vi "Create Engine Project.vi"(8 "error in":errorcluster, 10 "Custom Device Name":string, 11 "CDEW_MetaDataObj in":refnum<class "NIVS_CDEW_MetaDataObj.lvclass">) -> (0 "error out":errorcluster, 3 "CDEW_MetaDataObj out":refnum<class "NIVS_CDEW_MetaDataObj.lvclass">)   [LabVIEW 2026, in "NIVS_CDEW_MetaDataObj.lvclass"]
uses:
  NIVS_CDEW_MetaDataObj.lvclass
  Types/EngineProjectToolStates.ctl
  NIVS_CDEW_MetaDataObj.lvclass/NIVS_CDEW_MetaDataObj.ctl
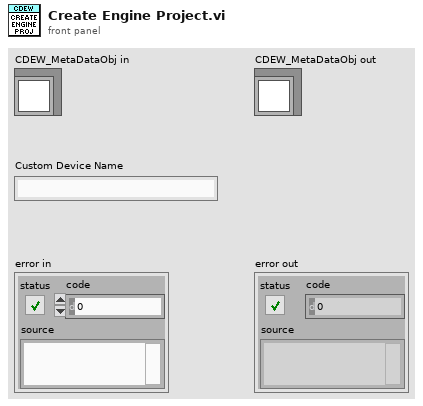
[diagram p1: front panel]
types:
  T1 = typedef "NIVS_CDEW_MetaDataObj.lvclass/EngineProjectToolStates.ctl" = enum16{"CreateEngineFolder", "CopyAndRenameEngineLVLIB", "UpdateLVLIBsInProject"}
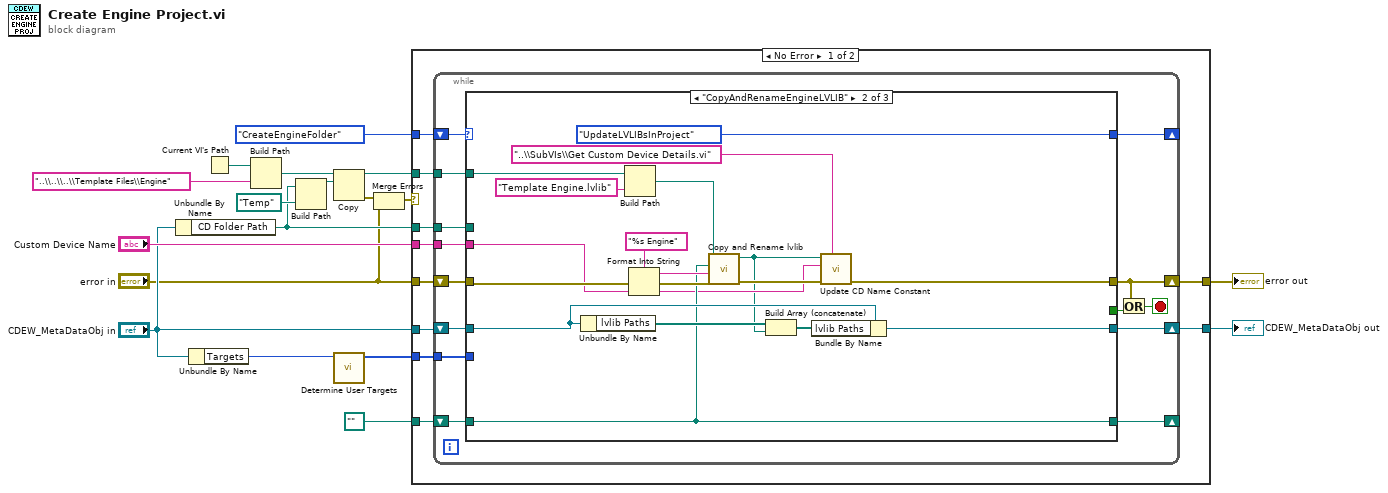
[diagram p0: block diagram]
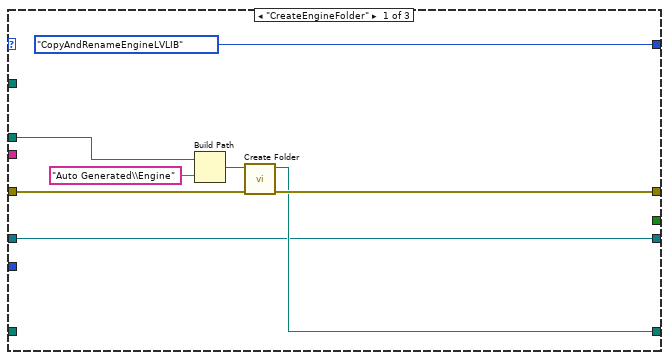
[diagram p2: hidden frame]
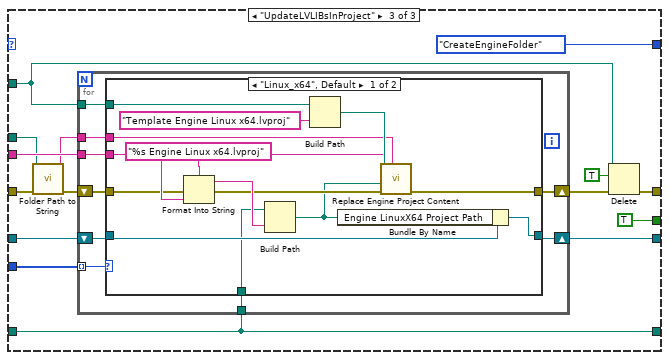
[diagram p3: hidden frame]
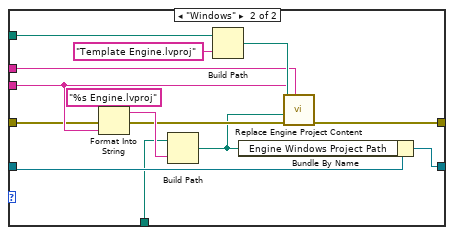
[diagram p4: hidden frame]
diagram:
  n1 = Unbundle By Name("CDEW_MetaDataObj in") -> ("CD Folder Path"=w8:path)
  n2 = Unbundle By Name("CDEW_MetaDataObj in") -> ("Targets"=w4:enum16{"Linux_x64", "Windows", "All"})
  n3 = Current VI's Path() -> (path=w16:path)
  n4 = Build Path(base path=w16, name or relative path="..\\..\\..\\Template Files\\Engine") -> (appended path=w11:path)
  n5 = Build Path(base path=w8, name or relative path=path "Temp") -> (appended path=w12:path)
  n6 = Copy(10:w12, 11:w11) -> (0:w3:errorcluster, 3:w10:path)  [unwired: 3 in, 1 out]
  n7 = call "Determine User Targets.vi"("Targets"=w4) -> ("User Configured Targets"=w5:enum16{"Linux_x64", "Windows", "All"}[])  [unwired: 10 in]
  n8 = Merge Errors(w3, "error in") -> (w1:errorcluster)
  n9 = case shown="No Error" w1 {
    selector: w1 -> [_ w120]
    tunnel: EngineProjectToolStates."CreateEngineFolder" -> [w28 _]
    tunnel: "Custom Device Name" -> [w27 _]
    tunnel: "error in" -> [w26 _]
    tunnel: [w25 w120] -> w14
    tunnel: w10 -> [w24 _]
    tunnel: [w23 w119] -> w9
    tunnel: w8 -> [w22 _]
    tunnel: path "" ("HarnessProjectPath") -> [w21 _]
    tunnel: "CDEW_MetaDataObj in" -> [w20 w119]
    tunnel: w5 -> [w19 _]
    frame No Error {
      n10 = while {
        shift-right: [w39] -> _
        shift-left: w28 -> [w42]
        tunnel: w27 -> [w41]
        tunnel: w24 -> [w40]
        shift-right: [w31] -> w23
        shift-left: w20 -> [w38]
        shift-right: [w36] -> w25
        shift-left: w26 -> [w37]
        shift-right: [w33] -> _
        shift-left: w21 -> [w32]
        tunnel: w22 -> [w30]
        tunnel: w19 -> [w29]
        stop <- w34 stop-if-true
        n11 = case shown="\"CopyAndRenameEngineLVLIB\"" w42 {
          tunnel: w41 -> [_ w53 w78]
          tunnel: w40 -> [_ w67 w72]
          tunnel: [EngineProjectToolStates."CopyAndRenameEngineLVLIB" EngineProjectToolStates."UpdateLVLIBsInProject" EngineProjectToolStates."CreateEngineFolder"] -> w39
          tunnel: [_ _ TRUE] -> w35
          tunnel: [w46 w57 w77] -> w31
          tunnel: w38 -> [w46 w59 w76]
          tunnel: [w48 w54 w80] -> w36
          tunnel: w37 -> [w49 w61 w69]
          tunnel: [w47 w56 w75] -> w33
          tunnel: w32 -> [_ w56 w75]
          tunnel: w30 -> [w45 _ w74]
          tunnel: w29 -> [_ _ w71]
          frame "CreateEngineFolder" {
            n12 = Build Path(base path=w45, name or relative path="Auto Generated\\Engine") -> (appended path=w44:path)
            n13 = call "Create Folder.vi"("error in"=w49, "Folder Path"=w44) -> ("error out"=w48:errorcluster, "Folder Path Out"=w47:path)  [unwired: 8 in]
          }
          frame "CopyAndRenameEngineLVLIB" {
            n14 = Unbundle By Name(w59) -> ("lvlib Paths"=w60:path[])
            n15 = Build Path(base path=w67, name or relative path="Template Engine.lvlib" ("string")) -> (appended path=w65:path)
            n16 = Format Into String(format string="%s Engine" ("string"), error in=w61, w53) -> (resulting string=w63:string, error out=w62:errorcluster)  [unwired: 1 in]
            n17 = call "Copy and Rename lvlib.vi"("error in"=w62, "New lvlib Name"=w63, "Destination Directory Path"=w56, "lvlib Path"=w65) -> ("error out"=w55:errorcluster, "New Library Path"=w52:path)  [unwired: 6 in]
            n18 = Build Array (concatenate)(w60, w52) -> (w58:path[])
            n19 = Bundle By Name(cluster=w59, "lvlib Paths"=w58) -> (w57:refnum<class "NIVS_CDEW_MetaDataObj.lvclass">)
            n20 = call "Update CD Name Constant.vi"("vi Name"="..\\SubVIs\\Get Custom Device Details.vi", "error in"=w55, "Custom Device Name"=w53, "lvlib Path"=w52) -> ("error out"=w54:errorcluster)  [unwired: 7 in]
          }
          frame "UpdateLVLIBsInProject" {
            n21 = call "Folder Path to String.vi"("error in"=w69, "CD Folder Path"=w74) -> ("error out"=w70:errorcluster, "Path as String"=w73:string)  [unwired: 8 in]
            n22 = for {
              tunnel: w72 -> [w91]
              tunnel: w78 -> [w90]
              tunnel: w75 -> [w86]
              tunnel: w73 -> [w85]
              shift-right: [w92] -> w81
              shift-left: w70 -> [w89]
              shift-right: [w88] -> w77
              shift-left: w76 -> [w87]
              tunnel: w71 -> [w84] mode=indexing
              n23 = case shown="\"Linux_x64\", Default" w84 {
                tunnel: [w103 w116] -> w92
                tunnel: w91 -> [w102 w115]
                tunnel: w90 -> [w101 w114]
                tunnel: w89 -> [w98 w111]
                tunnel: [w96 w109] -> w88
                tunnel: w87 -> [w95 w108]
                tunnel: w86 -> [w94 w107]
                tunnel: w85 -> [w93 w106]
                frame "Linux_x64", Default {
                  n24 = Format Into String(format string="%s Engine Linux x64.lvproj" ("Custom Device Name"), w101) -> (resulting string=w99:string)  [unwired: 2 in, 1 out]
                  n25 = Build Path(base path=w94, name or relative path=w99) -> (appended path=w97:path)
                  n26 = Build Path(base path=w102, name or relative path="Template Engine Linux x64.lvproj" ("Custom Device Name")) -> (appended path=w104:path)
                  n27 = Bundle By Name(cluster=w95, "Engine LinuxX64 Project Path"=w97) -> (w96:refnum<class "NIVS_CDEW_MetaDataObj.lvclass">)
                  n28 = call "Replace Engine Project Content.vi"("CDFolderPath String"=w93, "error in"=w98, "Custom Device Project Path"=w97, "CD Name"=w101, "Template Project path"=w104) -> ("error out"=w103:errorcluster)  [unwired: 6 in]
                }
                frame "Windows" {
                  n29 = Format Into String(format string="%s Engine.lvproj" ("Custom Device Name"), w114) -> (resulting string=w112:string)  [unwired: 2 in, 1 out]
                  n30 = Build Path(base path=w107, name or relative path=w112) -> (appended path=w110:path)
                  n31 = Build Path(base path=w115, name or relative path="Template Engine.lvproj" ("Custom Device Name")) -> (appended path=w117:path)
                  n32 = Bundle By Name(cluster=w108, "Engine Windows Project Path"=w110) -> (w109:refnum<class "NIVS_CDEW_MetaDataObj.lvclass">)
                  n33 = call "Replace Engine Project Content.vi"("CDFolderPath String"=w106, "error in"=w111, "Custom Device Project Path"=w110, "CD Name"=w114, "Template Project path"=w117) -> ("error out"=w116:errorcluster)  [unwired: 6 in]
                }
              }
            }
            n34 = Delete(path (use dialog)=w72, entire hierarchy (F)=TRUE, error in=w81) -> (error out=w80:errorcluster)  [unwired: 2 in, 2 out]
          }
        }
        n35 = Or(x=w36, y=w35) -> (x .or. y?=w34:bool)
      }
    }
    frame Error {
    }
  }
  "error out" <- w14
  "CDEW_MetaDataObj out" <- w9
